vi "svl_Check Data Valid [Integration].vi"(0 "signal in [X]":waveform(dbl)={"t0"=timestamp(0 s since 1904-01-01), "dt"=1.953125e-05, "Y"=[]}, 1 "reset (in)":bool, 5 "integration type":T1(ring)=enum."double integration", 7 "highpass cutoff frequency":dbl=1.0 format="%.2f", 11 "error in (no error)":errorcluster) -> (3 "reset (out)":bool, 4 "signal out [X]":waveform(dbl)={"t0"=timestamp(0 s since 1904-01-01), "dt"=1.953125e-05, "Y"=[]}, 6 "dup integration type":T1(ring)=enum."double integration", 8 "dup highpass cutoff frequency":dbl=1.0 format="%.2f", 15 "error out":errorcluster)   [LabVIEW 2017, in "SoundVib_Integration.lvlib"]
uses:
  <vilib>/addons/Sound and Vibration/svt_Integration/SoundVib_Integration.lvlib
  <vilib>/addons/_NISVFA/_Shared subVIs/Common/svc_Check for Waveform Parameter Continuity (no state).vi
  <vilib>/addons/_NISVFA/_Shared subVIs/Common/svc_Get SV Channel Info.vi
  <vilib>/addons/_NISVFA/_Shared subVIs/Common/svc_Engineering Units to Unit Label.vi
  <vilib>/addons/_NISVFA/_Shared subVIs/Common/svc_Unit Label to Engineering Units.vi
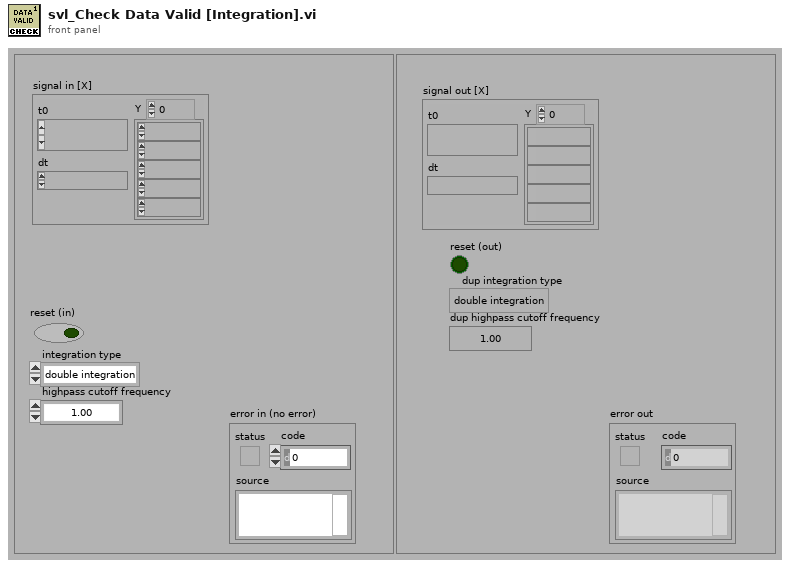
[diagram p1: front panel]
types:
  T1 = enum16{"single integration", "double integration"}
  T2 = cluster{"dt":bool, "t0 continuity":bool, "array length":bool, "channel info":bool, "name":bool}
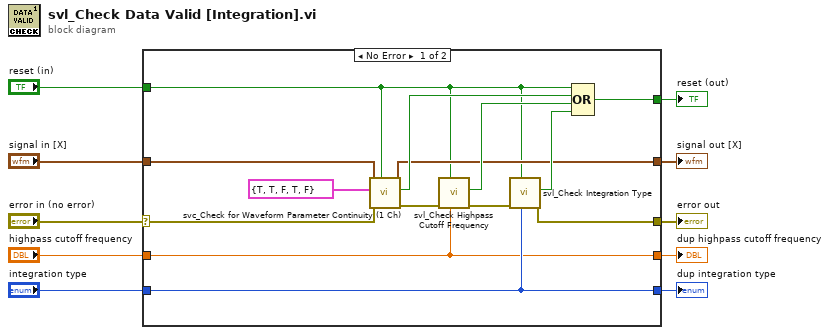
[diagram p0: block diagram]
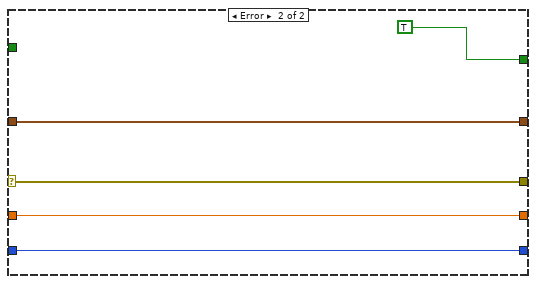
[diagram p2: hidden frame]
diagram:
  n1 = case shown="No Error" "error in (no error)" {
    selector: "error in (no error)" -> [w14 w29]
    tunnel: "signal in [X]" -> [w13 w28]
    tunnel: [w24 TRUE ("t0 changed")] -> w8
    tunnel: [w23 w29] -> w7
    tunnel: [w12 w28] -> w6
    tunnel: "reset (in)" -> [w11 _]
    tunnel: "highpass cutoff frequency" -> [w20 w26]
    tunnel: "integration type" -> [w21 w25]
    tunnel: [w20 w26] -> w2
    tunnel: [w21 w25] -> w1
    frame No Error {
      n2 = call <vilib>:"svc_Check for Waveform Parameter Continuity (1 Ch).vi"("restart averaging (F)"=w11, "error in (no error)"=w14, "checks for channel parameter change"=T2 {"dt"=TRUE, "t0 continuity"=TRUE, "array length"=FALSE, "channel info"=TRUE, "name"=FALSE}, "scaled signal [EU]"=w13) -> ("error out"=w17:errorcluster, "waveform parameter changed"=w15:bool, "dup scaled signal [EU]"=w12:waveform(dbl))  [unwired: 2 in, 3 out]
      n3 = call <vilib>:"svl_Check Highpass Cutoff Frequency.vi"("highpass cutoff frequency"=w20, "reset (in)"=w11, "error in (no error)"=w17) -> ("error out"=w18:errorcluster, "parameter has changed"=w19:bool)  [unwired: 7 in]
      n4 = call <vilib>:"svl_Check Integration Type.vi"("integration type"=w21, "reset (in)"=w11, "error in (no error)"=w18) -> ("error out"=w23:errorcluster, "parameter has changed"=w22:bool)  [unwired: 7 in]
      n5 = Compound Arithmetic op=OR(w11, w15, w19, w22) -> (w24:bool)
    }
    frame Error {
    }
  }
  "error out" <- w7
  "signal out [X]" <- w6
  "reset (out)" <- w8
  "dup integration type" <- w1
  "dup highpass cutoff frequency" <- w2
